vi "题目7.vi"() -> ()   [LabVIEW 2017]
uses:
  <vilib>/Utility/miscctls.llb/LVPositionTypeDef.ctl
  <vilib>/Utility/miscctls.llb/LVBoundsTypeDef.ctl
panel:
  in  "停止":bool
  in  "数值":dbl
  out "边界":T1
  in  "键选中":bool
  in  "可见":bool
  in  "禁用":T2(ring)
  in  "闪烁":bool
  in  "位置":T3
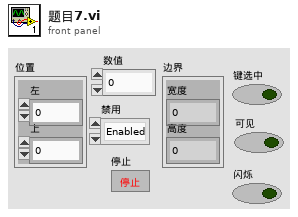
[diagram p1: front panel]
types:
  T1 = typedef "LVBoundsTypeDef.ctl" = cluster{"Width":u32, "Height":u32}
  T2 = enum8{"Enabled", "Disabled", "Disabled and Grayed Out"}
  T3 = typedef "LVPositionTypeDef.ctl" = cluster{"Left":i32, "Top":i32}
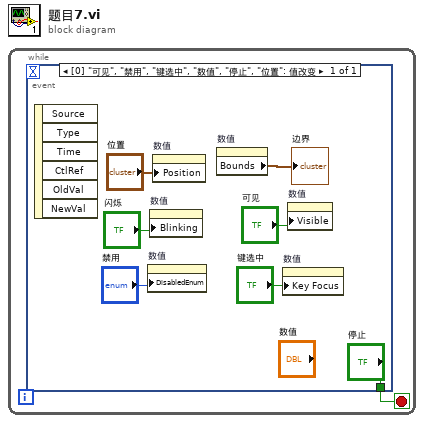
[diagram p0: block diagram]
diagram:
  n1 = while {
    stop <- w1 stop-if-true
    n2 = event shown="[0] \"可见\", \"禁用\", \"键选中\", \"数值\", \"停止\", \"位置\": 值改变" {
      selector: _ -> [_]
      dyn-events: _ -> [_]
      timeout: _ -> [_]
      tunnel: ["停止"] -> w1
      event "可见", "禁用", "键选中", "数值", "停止": Value Change {
        n3 = event-data() -> ()  [unwired: 1 in, 6 out]
        n4 = property on="数值" class="DigNum (严格)"("DisabledEnum"="禁用") -> ()  [unwired: 2 in, 2 out]
        n5 = property on="数值" class="DigNum (严格)"("Blinking"="闪烁") -> ()  [unwired: 2 in, 2 out]
        n6 = property on="数值" class="DigNum (严格)"("Position"="位置") -> ()  [unwired: 2 in, 2 out]
        n7 = property on="数值" class="DigNum (严格)"() -> ("Bounds"=→"边界":T1)  [unwired: 2 in, 2 out]
        n8 = property on="数值" class="DigNum (严格)"("Key Focus"="键选中") -> ()  [unwired: 2 in, 2 out]
        n9 = property on="数值" class="DigNum (严格)"("Visible"="可见") -> ()  [unwired: 2 in, 2 out]
      }
    }
  }
